vi "OE2012&OE2022_Ethernet_Query Data.vi"(0 "Connection ID in":refnum<k5>, 9 "Timeout":u32=40, 11 "Error in (no error)":errorcluster caption="error out（no error）") -> (1 "ChannelA_Configure":T1={"InputSource"=0, "InputCoupling"=0, "Input Range"=0, "Time Constant(s) "=0.0, "Low Pass Filter Slope "=1, "InputGround"=0, "Enable Sync Filter"=0, "Reference Source"=0, "External Ref Trigger"=0, "Phase0 (degree)"=0.0, "Phase1 (degree)"=0.0, "Phase2 (degree)"=0.0, "Phase3 (degree)"=0.0, "Phase4 (degree)"=0.0, "Phase5 (degree)"=0.0, "Phase6 (degree)"=0.0, "Phase7 (degree)"=0.0, "Osc1 Frequency(Hz)"=0.0, "Osc2 Frequency(Hz)"=0.0, "Demodulator type_1"=0, "Demodulator type_2"=0, "Demodulator type_3"=0, "Demodulator type_4"=0, "Demodulator type_5"=0, "Demodulator type_6"=0, "Demodulator type_7"=0, "Demodulator type_8"=0, "Demodulator harm_1"=0, "Demodulator harm_2"=0, "Demodulator harm_3"=0, "Demodulator harm_4"=0, "Demodulator harm_5"=0, "Demodulator harm_6"=0, "Demodulator harm_7"=0, "Demodulator harm_8"=0, "Demodulator freq_1"=0.0, "Demodulator freq_2"=0.0, "Demodulator freq_3"=0.0, "Demodulator freq_4"=0.0, "Demodulator freq_5"=0.0, "Demodulator freq_6"=0.0, "Demodulator freq_7"=0.0, "Demodulator freq_8"=0.0, "SineOut Mode"=0, "SineOut TTL Switch"=0, "Sine Output Amplitude(V)"=0.0, "Sine Output Offest (V)"=0.0, "CH1_Source"=3, "CH2_Source"=3, "CH3_Source"=3, "CH4_Source"=3, "CH1 AUX OUT"=0.0, "CH2 AUX OUT"=0.0, "CH3 AUX OUT"=0.0, "CH4 AUX OUT"=0.0, "CH1 Offset(%)"=0.0, "CH2 Offset(%)"=0.0, "CH3 Offset(%)"=0.0, "CH4 Offset(%)"=0.0, "CH1 Expand"=0.0, "CH2 Expand"=0.0, "CH3 Expand"=0.0, "CH4 Expand"=0.0, "CH1_Sensitivity "=24, "CH2_Sensitivity "=24, "CH3_Sensitivity"=24, "CH4_Sensitivity"=24, "Input ovld state"=FALSE, "Gain ovld state"=FALSE, "PLL state"=FALSE} {"CH4_Sensitivity" items=["1 nV/fA", "2 nV/fA", "5 nV/fA", "10 nV/fA", "20 nV/fA", "50 nV/fA", "100 nV/fA", "200 nV/fA", "500 nV/fA", "1 uV/pA", "2 uV/pA", "5 uV/pA", "10 uV/pA", "20 uV/pA", "50 uV/pA", "100 uV/pA", "200 uV/pA", "500 uV/pA", "1 mV/nA", "2 mV/nA", "5 mV/nA", "10 mV/nA", "20 mV/nA", "50 mV/nA", "100 mV/nA", "200 mV/nA", "500 mV/nA", "1 V/uA", "2 V/uA", "5 V/uA"]; "CH3_Sensitivity" items=["1 nV/fA", "2 nV/fA", "5 nV/fA", "10 nV/fA", "20 nV/fA", "50 nV/fA", "100 nV/fA", "200 nV/fA", "500 nV/fA", "1 uV/pA", "2 uV/pA", "5 uV/pA", "10 uV/pA", "20 uV/pA", "50 uV/pA", "100 uV/pA", "200 uV/pA", "500 uV/pA", "1 mV/nA", "2 mV/nA", "5 mV/nA", "10 mV/nA", "20 mV/nA", "50 mV/nA", "100 mV/nA", "200 mV/nA", "500 mV/nA", "1 V/uA", "2 V/uA", "5 V/uA"]; "CH2_Sensitivity" items=["1 nV/fA", "2 nV/fA", "5 nV/fA", "10 nV/fA", "20 nV/fA", "50 nV/fA", "100 nV/fA", "200 nV/fA", "500 nV/fA", "1 uV/pA", "2 uV/pA", "5 uV/pA", "10 uV/pA", "20 uV/pA", "50 uV/pA", "100 uV/pA", "200 uV/pA", "500 uV/pA", "1 mV/nA", "2 mV/nA", "5 mV/nA", "10 mV/nA", "20 mV/nA", "50 mV/nA", "100 mV/nA", "200 mV/nA", "500 mV/nA", "1 V/uA", "2 V/uA", "5 V/uA"]; "CH1_Sensitivity" items=["1 nV/fA", "2 nV/fA", "5 nV/fA", "10 nV/fA", "20 nV/fA", "50 nV/fA", "100 nV/fA", "200 nV/fA", "500 nV/fA", "1 uV/pA", "2 uV/pA", "5 uV/pA", "10 uV/pA", "20 uV/pA", "50 uV/pA", "100 uV/pA", "200 uV/pA", "500 uV/pA", "1 mV/nA", "2 mV/nA", "5 mV/nA", "10 mV/nA", "20 mV/nA", "50 mV/nA", "100 mV/nA", "200 mV/nA", "500 mV/nA", "1 V/uA", "2 V/uA", "5 V/uA"]; "CH4_Source" items=["DC OUT", "X-Demod1", "Y-Demod1", "R-Demod1", "Theta-Demod1", "X-Demod2", "Y-Demod2", "R-Demod2", "Theta-Demod2", "X-Demod3", "Y-Demod3", "R-Demod3", "Theta-Demod3", "X-Demod4", "Y-Demod4", "R-Demod4", "Theta-Demod4", "X-Demod5", "Y-Demod5", "R-Demod5", "Theta-Demod5", "X-Demod6", "Y-Demod6", "R-Demod6", "Theta-Demod6", "X-Demod7", "Y-Demod7", "R-Demod7", "Theta-Demod7", "X-Demod8", "Y-Demod8", "R-Demod8", "Theta-Demod8", "AUXIN1", "AUXIN2", "AUXIN3", "AUXIN4"]; "CH3_Source" items=["DC OUT", "X-Demod1", "Y-Demod1", "R-Demod1", "Theta-Demod1", "X-Demod2", "Y-Demod2", "R-Demod2", "Theta-Demod2", "X-Demod3", "Y-Demod3", "R-Demod3", "Theta-Demod3", "X-Demod4", "Y-Demod4", "R-Demod4", "Theta-Demod4", "X-Demod5", "Y-Demod5", "R-Demod5", "Theta-Demod5", "X-Demod6", "Y-Demod6", "R-Demod6", "Theta-Demod6", "X-Demod7", "Y-Demod7", "R-Demod7", "Theta-Demod7", "X-Demod8", "Y-Demod8", "R-Demod8", "Theta-Demod8", "AUXIN1", "AUXIN2", "AUXIN3", "AUXIN4"]; "CH2_Source" items=["DC OUT", "X-Demod1", "Y-Demod1", "R-Demod1", "Theta-Demod1", "X-Demod2", "Y-Demod2", "R-Demod2", "Theta-Demod2", "X-Demod3", "Y-Demod3", "R-Demod3", "Theta-Demod3", "X-Demod4", "Y-Demod4", "R-Demod4", "Theta-Demod4", "X-Demod5", "Y-Demod5", "R-Demod5", "Theta-Demod5", "X-Demod6", "Y-Demod6", "R-Demod6", "Theta-Demod6", "X-Demod7", "Y-Demod7", "R-Demod7", "Theta-Demod7", "X-Demod8", "Y-Demod8", "R-Demod8", "Theta-Demod8", "AUXIN1", "AUXIN2", "AUXIN3", "AUXIN4"]; "CH1_Source" items=["DC OUT", "X-Demod1", "Y-Demod1", "R-Demod1", "Theta-Demod1", "X-Demod2", "Y-Demod2", "R-Demod2", "Theta-Demod2", "X-Demod3", "Y-Demod3", "R-Demod3", "Theta-Demod3", "X-Demod4", "Y-Demod4", "R-Demod4", "Theta-Demod4", "X-Demod5", "Y-Demod5", "R-Demod5", "Theta-Demod5", "X-Demod6", "Y-Demod6", "R-Demod6", "Theta-Demod6", "X-Demod7", "Y-Demod7", "R-Demod7", "Theta-Demod7", "X-Demod8", "Y-Demod8", "R-Demod8", "Theta-Demod8", "AUXIN1", "AUXIN2", "AUXIN3", "AUXIN4"]; "SineOut TTL Switch" items=["OFF", "On"]; "SineOut Mode" items=["OFF", "On"]; "Demodulator type_8" items=["Osc1", "Osc2", "Harm", "Arb_Freq"]; "Demodulator type_7" items=["Osc1", "Osc2", "Harm", "Arb_Freq"]; "Demodulator type_6" items=["Osc1", "Osc2", "Harm", "Arb_Freq"]; "Demodulator type_5" items=["Osc1", "Osc2", "Harm", "Arb_Freq"]; "Demodulator type_4" items=["Osc1", "Osc2", "Harm", "Arb_Freq"]; "Demodulator type_3" items=["Osc1", "Osc2", "Harm", "Arb_Freq"]; "Demodulator type_2" items=["Osc1", "Osc2", "Harm", "Arb_Freq"]; "Demodulator type_1" items=["Osc1", "Osc2", "Harm", "Arb_Freq"]; "External Ref Trigger" items=["TTL Rising Edge", "TTL Fallling Edge", "Sine Zero Crossing"]; "Reference Source" items=["External", "Internal"]; "Enable Sync Filter" items=["OFF", "ON"]; "InputGround" items=["FLoat", "Ground"]; "Low Pass Filter Slope" items=["6 dB/oct", "12 dB/oct", "18 db/oct", "24 dB/oct", "30 dB/oct", "36 dB/oct", "42 dB/oct", "48 dB/oct"]; "Input Range" items=["2V", "500mV", "200mV", "50mV", "20mV", "5mV", "2mV"]; "InputCoupling" items=["AC", "DC"]; "InputSource" items=["A", "A-B", "Current"]}, 3 "Buffer Count":u8, 4 "Connection ID out":refnum<k5>, 6 "Parameter Values":T2, 8 "Total Date Array":dbl[][](array[numeric]), 10 "Output String":string, 12 "ChannelB_Configure":T1={"InputSource"=0, "InputCoupling"=0, "Input Range"=0, "Time Constant(s) "=0.0, "Low Pass Filter Slope "=1, "InputGround"=0, "Enable Sync Filter"=0, "Reference Source"=0, "External Ref Trigger"=0, "Phase0 (degree)"=0.0, "Phase1 (degree)"=0.0, "Phase2 (degree)"=0.0, "Phase3 (degree)"=0.0, "Phase4 (degree)"=0.0, "Phase5 (degree)"=0.0, "Phase6 (degree)"=0.0, "Phase7 (degree)"=0.0, "Osc1 Frequency(Hz)"=0.0, "Osc2 Frequency(Hz)"=0.0, "Demodulator type_1"=0, "Demodulator type_2"=0, "Demodulator type_3"=0, "Demodulator type_4"=0, "Demodulator type_5"=0, "Demodulator type_6"=0, "Demodulator type_7"=0, "Demodulator type_8"=0, "Demodulator harm_1"=0, "Demodulator harm_2"=0, "Demodulator harm_3"=0, "Demodulator harm_4"=0, "Demodulator harm_5"=0, "Demodulator harm_6"=0, "Demodulator harm_7"=0, "Demodulator harm_8"=0, "Demodulator freq_1"=0.0, "Demodulator freq_2"=0.0, "Demodulator freq_3"=0.0, "Demodulator freq_4"=0.0, "Demodulator freq_5"=0.0, "Demodulator freq_6"=0.0, "Demodulator freq_7"=0.0, "Demodulator freq_8"=0.0, "SineOut Mode"=0, "SineOut TTL Switch"=0, "Sine Output Amplitude(V)"=0.0, "Sine Output Offest (V)"=0.0, "CH1_Source"=3, "CH2_Source"=3, "CH3_Source"=3, "CH4_Source"=3, "CH1 AUX OUT"=0.0, "CH2 AUX OUT"=0.0, "CH3 AUX OUT"=0.0, "CH4 AUX OUT"=0.0, "CH1 Offset(%)"=0.0, "CH2 Offset(%)"=0.0, "CH3 Offset(%)"=0.0, "CH4 Offset(%)"=0.0, "CH1 Expand"=0.0, "CH2 Expand"=0.0, "CH3 Expand"=0.0, "CH4 Expand"=0.0, "CH1_Sensitivity "=24, "CH2_Sensitivity "=24, "CH3_Sensitivity"=24, "CH4_Sensitivity"=24, "Input ovld state"=FALSE, "Gain ovld state"=FALSE, "PLL state"=FALSE} {"CH4_Sensitivity" items=["1 nV/fA", "2 nV/fA", "5 nV/fA", "10 nV/fA", "20 nV/fA", "50 nV/fA", "100 nV/fA", "200 nV/fA", "500 nV/fA", "1 uV/pA", "2 uV/pA", "5 uV/pA", "10 uV/pA", "20 uV/pA", "50 uV/pA", "100 uV/pA", "200 uV/pA", "500 uV/pA", "1 mV/nA", "2 mV/nA", "5 mV/nA", "10 mV/nA", "20 mV/nA", "50 mV/nA", "100 mV/nA", "200 mV/nA", "500 mV/nA", "1 V/uA", "2 V/uA", "5 V/uA"]; "CH3_Sensitivity" items=["1 nV/fA", "2 nV/fA", "5 nV/fA", "10 nV/fA", "20 nV/fA", "50 nV/fA", "100 nV/fA", "200 nV/fA", "500 nV/fA", "1 uV/pA", "2 uV/pA", "5 uV/pA", "10 uV/pA", "20 uV/pA", "50 uV/pA", "100 uV/pA", "200 uV/pA", "500 uV/pA", "1 mV/nA", "2 mV/nA", "5 mV/nA", "10 mV/nA", "20 mV/nA", "50 mV/nA", "100 mV/nA", "200 mV/nA", "500 mV/nA", "1 V/uA", "2 V/uA", "5 V/uA"]; "CH2_Sensitivity" items=["1 nV/fA", "2 nV/fA", "5 nV/fA", "10 nV/fA", "20 nV/fA", "50 nV/fA", "100 nV/fA", "200 nV/fA", "500 nV/fA", "1 uV/pA", "2 uV/pA", "5 uV/pA", "10 uV/pA", "20 uV/pA", "50 uV/pA", "100 uV/pA", "200 uV/pA", "500 uV/pA", "1 mV/nA", "2 mV/nA", "5 mV/nA", "10 mV/nA", "20 mV/nA", "50 mV/nA", "100 mV/nA", "200 mV/nA", "500 mV/nA", "1 V/uA", "2 V/uA", "5 V/uA"]; "CH1_Sensitivity" items=["1 nV/fA", "2 nV/fA", "5 nV/fA", "10 nV/fA", "20 nV/fA", "50 nV/fA", "100 nV/fA", "200 nV/fA", "500 nV/fA", "1 uV/pA", "2 uV/pA", "5 uV/pA", "10 uV/pA", "20 uV/pA", "50 uV/pA", "100 uV/pA", "200 uV/pA", "500 uV/pA", "1 mV/nA", "2 mV/nA", "5 mV/nA", "10 mV/nA", "20 mV/nA", "50 mV/nA", "100 mV/nA", "200 mV/nA", "500 mV/nA", "1 V/uA", "2 V/uA", "5 V/uA"]; "CH4_Source" items=["DC OUT", "X-Demod1", "Y-Demod1", "R-Demod1", "Theta-Demod1", "X-Demod2", "Y-Demod2", "R-Demod2", "Theta-Demod2", "X-Demod3", "Y-Demod3", "R-Demod3", "Theta-Demod3", "X-Demod4", "Y-Demod4", "R-Demod4", "Theta-Demod4", "X-Demod5", "Y-Demod5", "R-Demod5", "Theta-Demod5", "X-Demod6", "Y-Demod6", "R-Demod6", "Theta-Demod6", "X-Demod7", "Y-Demod7", "R-Demod7", "Theta-Demod7", "X-Demod8", "Y-Demod8", "R-Demod8", "Theta-Demod8", "AUXIN1", "AUXIN2", "AUXIN3", "AUXIN4"]; "CH3_Source" items=["DC OUT", "X-Demod1", "Y-Demod1", "R-Demod1", "Theta-Demod1", "X-Demod2", "Y-Demod2", "R-Demod2", "Theta-Demod2", "X-Demod3", "Y-Demod3", "R-Demod3", "Theta-Demod3", "X-Demod4", "Y-Demod4", "R-Demod4", "Theta-Demod4", "X-Demod5", "Y-Demod5", "R-Demod5", "Theta-Demod5", "X-Demod6", "Y-Demod6", "R-Demod6", "Theta-Demod6", "X-Demod7", "Y-Demod7", "R-Demod7", "Theta-Demod7", "X-Demod8", "Y-Demod8", "R-Demod8", "Theta-Demod8", "AUXIN1", "AUXIN2", "AUXIN3", "AUXIN4"]; "CH2_Source" items=["DC OUT", "X-Demod1", "Y-Demod1", "R-Demod1", "Theta-Demod1", "X-Demod2", "Y-Demod2", "R-Demod2", "Theta-Demod2", "X-Demod3", "Y-Demod3", "R-Demod3", "Theta-Demod3", "X-Demod4", "Y-Demod4", "R-Demod4", "Theta-Demod4", "X-Demod5", "Y-Demod5", "R-Demod5", "Theta-Demod5", "X-Demod6", "Y-Demod6", "R-Demod6", "Theta-Demod6", "X-Demod7", "Y-Demod7", "R-Demod7", "Theta-Demod7", "X-Demod8", "Y-Demod8", "R-Demod8", "Theta-Demod8", "AUXIN1", "AUXIN2", "AUXIN3", "AUXIN4"]; "CH1_Source" items=["DC OUT", "X-Demod1", "Y-Demod1", "R-Demod1", "Theta-Demod1", "X-Demod2", "Y-Demod2", "R-Demod2", "Theta-Demod2", "X-Demod3", "Y-Demod3", "R-Demod3", "Theta-Demod3", "X-Demod4", "Y-Demod4", "R-Demod4", "Theta-Demod4", "X-Demod5", "Y-Demod5", "R-Demod5", "Theta-Demod5", "X-Demod6", "Y-Demod6", "R-Demod6", "Theta-Demod6", "X-Demod7", "Y-Demod7", "R-Demod7", "Theta-Demod7", "X-Demod8", "Y-Demod8", "R-Demod8", "Theta-Demod8", "AUXIN1", "AUXIN2", "AUXIN3", "AUXIN4"]; "SineOut TTL Switch" items=["OFF", "On"]; "SineOut Mode" items=["OFF", "On"]; "Demodulator type_8" items=["Osc1", "Osc2", "Harm", "Arb_Freq"]; "Demodulator type_7" items=["Osc1", "Osc2", "Harm", "Arb_Freq"]; "Demodulator type_6" items=["Osc1", "Osc2", "Harm", "Arb_Freq"]; "Demodulator type_5" items=["Osc1", "Osc2", "Harm", "Arb_Freq"]; "Demodulator type_4" items=["Osc1", "Osc2", "Harm", "Arb_Freq"]; "Demodulator type_3" items=["Osc1", "Osc2", "Harm", "Arb_Freq"]; "Demodulator type_2" items=["Osc1", "Osc2", "Harm", "Arb_Freq"]; "Demodulator type_1" items=["Osc1", "Osc2", "Harm", "Arb_Freq"]; "External Ref Trigger" items=["TTL Rising Edge", "TTL Fallling Edge", "Sine Zero Crossing"]; "Reference Source" items=["External", "Internal"]; "Enable Sync Filter" items=["OFF", "ON"]; "InputGround" items=["FLoat", "Ground"]; "Low Pass Filter Slope" items=["6 dB/oct", "12 dB/oct", "18 db/oct", "24 dB/oct", "30 dB/oct", "36 dB/oct", "42 dB/oct", "48 dB/oct"]; "Input Range" items=["2V", "500mV", "200mV", "50mV", "20mV", "5mV", "2mV"]; "InputCoupling" items=["AC", "DC"]; "InputSource" items=["A", "A-B", "Current"]}, 13 "Trig_Count":u8[](array[numeric]), 14 "PLL&Overload":T3, 15 "Error out":errorcluster caption="error out")   [LabVIEW 2011]
panel:
  out "Read Buffer":string
  in  "buffer":string
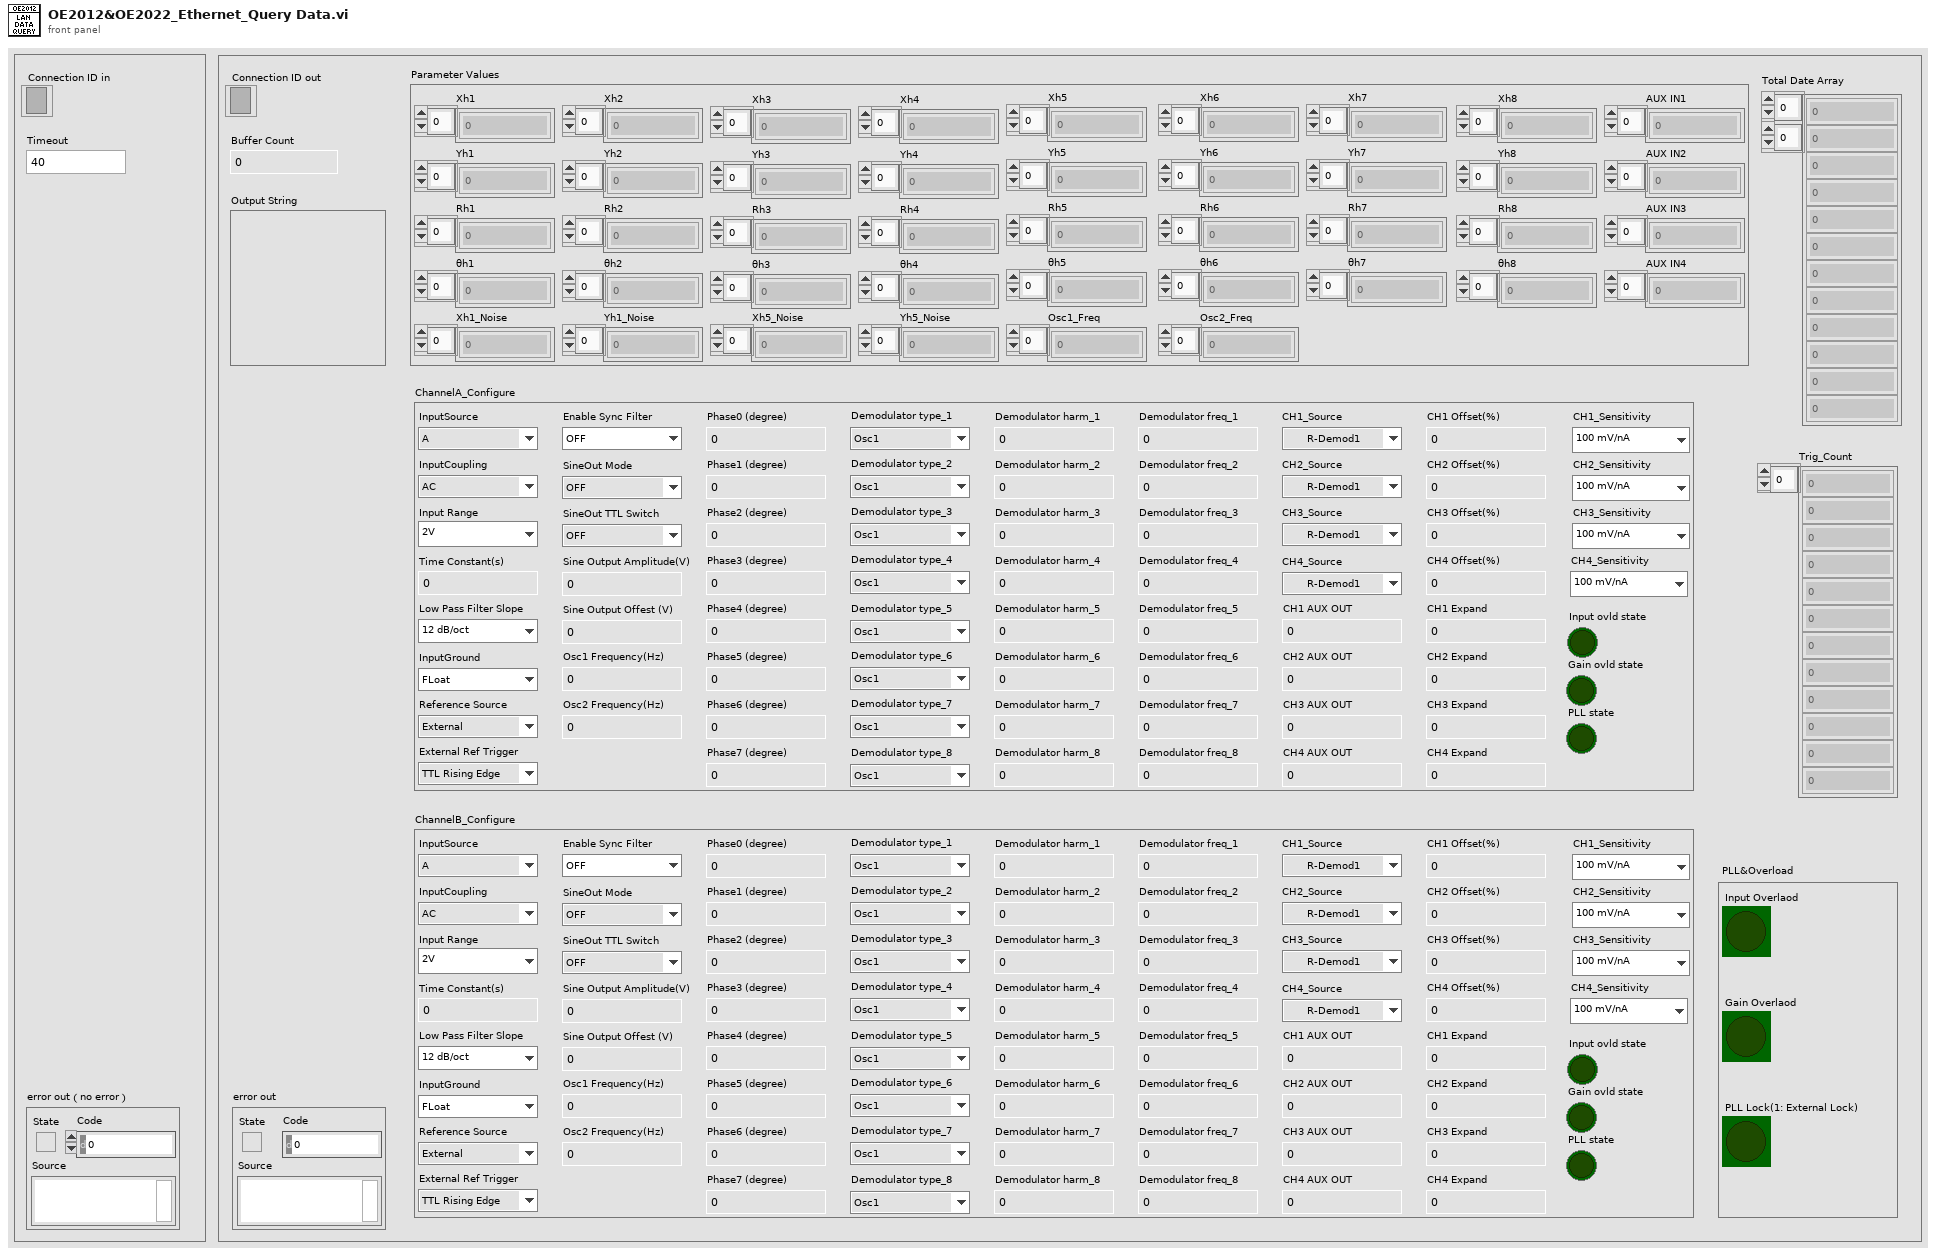
[diagram p1: front panel]
types:
  T1 = cluster{"InputSource":u8, "InputCoupling":u8, "Input Range":u8, "Time Constant(s) ":dbl, "Low Pass Filter Slope ":u8, "InputGround":u8, "Enable Sync Filter":u8, "Reference Source":u8, "External Ref Trigger":u8, "Phase0 (degree)":sgl, "Phase1 (degree)":sgl, "Phase2 (degree)":sgl, "Phase3 (degree)":sgl, "Phase4 (degree)":sgl, "Phase5 (degree)":sgl, "Phase6 (degree)":sgl, "Phase7 (degree)":sgl, "Osc1 Frequency(Hz)":dbl, "Osc2 Frequency(Hz)":dbl, "Demodulator type_1":u8, "Demodulator type_2":u8, "Demodulator type_3":u8, "Demodulator type_4":u8, "Demodulator type_5":u8, "Demodulator type_6":u8, "Demodulator type_7":u8, "Demodulator type_8":u8, "Demodulator harm_1":u16, "Demodulator harm_2":u16, "Demodulator harm_3":u16, "Demodulator harm_4":u16, "Demodulator harm_5":u16, "Demodulator harm_6":u16, "Demodulator harm_7":u16, "Demodulator harm_8":u16, "Demodulator freq_1":dbl, "Demodulator freq_2":dbl, "Demodulator freq_3":dbl, "Demodulator freq_4":dbl, "Demodulator freq_5":dbl, "Demodulator freq_6":dbl, "Demodulator freq_7":dbl, "Demodulator freq_8":dbl, "SineOut Mode":u8, "SineOut TTL Switch":u8, "Sine Output Amplitude(V)":dbl, "Sine Output Offest (V)":dbl, "CH1_Source":u8, "CH2_Source":u8, "CH3_Source":u8, "CH4_Source":u8, "CH1 AUX OUT":dbl, "CH2 AUX OUT":dbl, "CH3 AUX OUT":dbl, "CH4 AUX OUT":dbl, "CH1 Offset(%)":dbl, "CH2 Offset(%)":dbl, "CH3 Offset(%)":dbl, "CH4 Offset(%)":dbl, "CH1 Expand":dbl, "CH2 Expand":dbl, "CH3 Expand":dbl, "CH4 Expand":dbl, "CH1_Sensitivity ":u8, "CH2_Sensitivity ":u8, "CH3_Sensitivity":u8, "CH4_Sensitivity":u8, "Input ovld state":bool, "Gain ovld state":bool, "PLL state":bool}
  T2 = cluster{"Xh1":dbl[], "Yh1":dbl[], "Rh1":dbl[], "θh1":dbl[], "Xh1_Noise":dbl[], "Yh1_Noise":dbl[], "Xh2":dbl[], "Yh2":dbl[], "Rh2":dbl[], "θh2":dbl[], "Xh3":dbl[], "Yh3":dbl[], "Rh3":dbl[], "θh3":dbl[], "Xh4":dbl[], "Yh4":dbl[], "Rh4":dbl[], "θh4":dbl[], "Xh5":dbl[], "Yh5":dbl[], "Rh5":dbl[], "θh5":dbl[], "Xh5_Noise":dbl[], "Yh5_Noise":dbl[], "Xh6":dbl[], "Yh6":dbl[], "Rh6":dbl[], "θh6":dbl[], "Xh7":dbl[], "Yh7":dbl[], "Rh7":dbl[], "θh7":dbl[], "Xh8":dbl[], "Yh8":dbl[], "Rh8":dbl[], "θh8":dbl[], "Osc1_Freq":dbl[], "Osc2_Freq":dbl[], "AUX IN1":dbl[], "AUX IN2":dbl[], "AUX IN3":dbl[], "AUX IN4":dbl[]}
  T3 = cluster{"Input Overlaod":bool, "Gain Overlaod":bool, "PLL Lock(1: External Lock)":bool}
  T4 = cluster{"Xh1":dbl[], "Yh1":dbl[], "Rh1":dbl[], "θh1":dbl[], "Xh1_Noise":dbl[], "Yh1_Noise":dbl[], "Xh2":dbl[], "Yh2":dbl[], "Rh2":dbl[], "θh2":dbl[], "Xh3":dbl[], "Yh3":dbl[], "Rh3":dbl[], "θh3":dbl[], "Xh4":dbl[], "Yh4":dbl[], "Rh4":dbl[], "θh4":dbl[], "Xh5":dbl[], "Yh5":dbl[], "Rh5":dbl[], "θh5":dbl[], "Xh5_Noise":dbl[], "Yh5_Noise":dbl[], "Xh6":dbl[], "Yh6":dbl[], "Rh6":dbl[], "θh6":dbl[], "Xh7":dbl[], "Yh7":dbl[], "Rh7":dbl[], "θh7":dbl[], "Xh8":dbl[], "Yh8":dbl[], "Rh8":dbl[], "θh8":dbl[], "Osc1_Freq":dbl[], "Osc2_Freq":dbl[], "AUXOUT1":dbl[], "AUXOUT2":dbl[], "AUXOUT3":dbl[], "AUXOUT4":dbl[]}
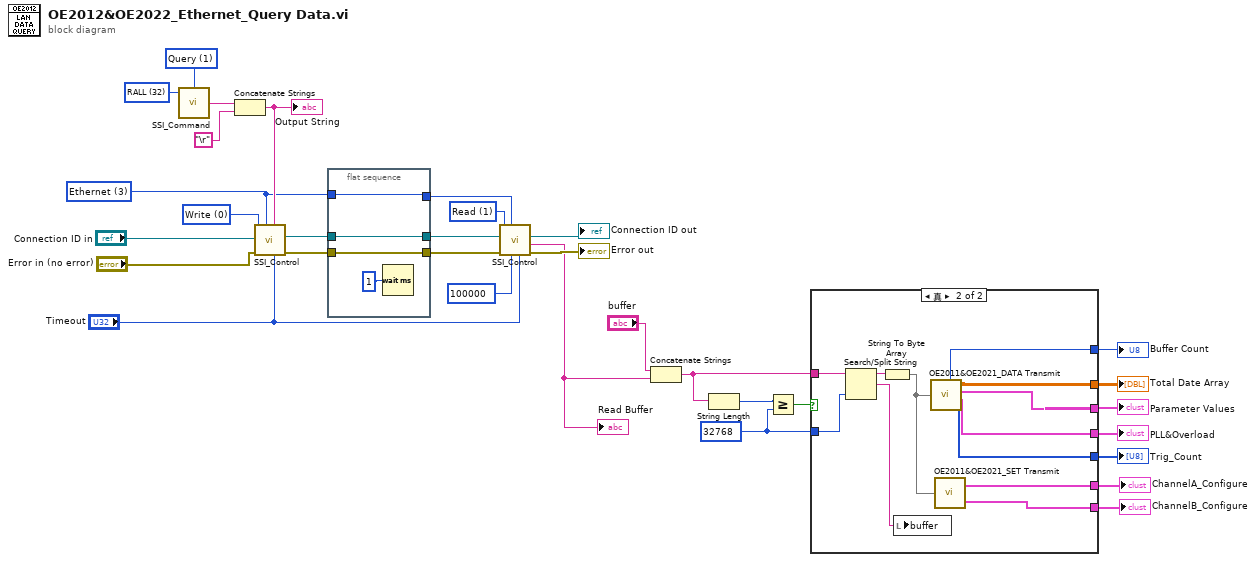
[diagram p0: block diagram]
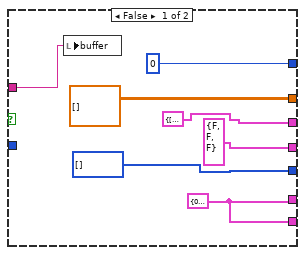
[diagram p2: hidden frame]
diagram:
  w9 = 32768 ("y")
  w26 = u16 3 items=["USB", "RS232", "GPIB", "Ethernet"] ("Remote Mode")
  w22 = u16 32 items=["ISRC", "IGND", "ICPL", "ILIN", "PHAS", "FMOD", "RSLP", "FREQ", "SWPT", "SLLM", "SULM", "SSLL", "SSLG", "STLM", "SWRM", "IRNG", "SENS", "RMOD", "OFLT", "OFSL", "SYNC", "DMOD", "HARM", "DARB", "SWVT", "SLVL", "SVLL", "SVUL", "SVSL", "SVSG", "SVTM", "SVRM", "RALL", "SNAP", "OUTP", "OAUX", "COUT", "CAUX", "COFP", "CEXP", "FPOP", "OEXP", "*IDN", "*RST", "OVLD", "INOV", "GNOV", "*PLL", "SSET", "RSET", "AGAN", "APHS", "ARSV", "ASCL", "EQCD", "EQCS", "SPED", "SRAT", "SLEN", "SSLE", "STRG", "SPRM", "STRD", "PAUS", "RSET", "SPTS", "TRCA", "TEMP", "RSTU", "INHZ", "DEQU", "SADD", "ARNG", "CSPE", "ISRCD", "IGNDD", "ICPLD", "ILIND", "PHASD", "FMODD", "RSLPD", "FREQD", "SWPTD", "SLLMD", "SULMD", "SSLLD", "SSLGD", "STLMD", "SWRMD", "SENSD", "RMODD", "OFLTD", "OFSLD", "SYNCD", "HARMD", "EQCDD", "EQCSD", "SNAPD", "OUTPD", "SWVTD", "SLVLD", "SVLLD", "SVULD", "SVSLD", "SVSGD", "SVTMD", "SVRMD", "SVDCD", "ARSVD", "AGAND", "APHSD", "ASCLD", "FPOPD", "CAUXD", "OEXPD", "SPEDD", "SRATD", "SLEND", "SSLED", "STRGD", "SPRMD", "STRDD", "PAUSD", "RESTD", "SPTSD", "TRCAD", "*IDND", "*RSTD", "INOVD", "GNOVD", "*PLLD", "SSETD", "RSETD", "RALLD"] ("Command Type")
  w20 = u16 1 items=["Set", "Query"] ("Opera")
  w29 = u16 1 items=["Write", "Read"] ("Control")
  w32 = u16 0 items=["Write", "Read"] ("Control")
  n1 = call "SSI_Command.vi"("Opera"=w20, "Command Type"=w22) -> ("Output string"=w21:string)  [unwired: 2 in]
  n2 = Concatenate Strings(w21, "\r") -> (w27:string)
  "Output String" <- w27
  n3 = call "SSI_Control.vi"("Tineout"="Timeout", "Write Buffer"=w27, "Remote Mode"=w26, "Error in (no error)"="Error in (no error)", "Control"=w32, "Connection ID in"="Connection ID in") -> ("Error out"=w31:errorcluster, "Connection ID out"=w6:refnum<k5>)  [unwired: 2 in, 2 out]
  n4 = flat-sequence {
    tunnel: w31 -> [w36]
    tunnel: [w36] -> w30
    tunnel: [w34] -> w28
    tunnel: w26 -> [w34]
    tunnel: w6 -> [w33]
    tunnel: [w33] -> w5
    frame #0 {
      n5 = Wait (ms)(milliseconds to wait=u32 1 ("等待时间（毫秒）")) -> ()  [unwired: 1 out]
    }
  }
  n6 = call "SSI_Control.vi"("Tineout"="Timeout", "Number of bytes"=u32 100000, "Remote Mode"=w28, "Error in (no error)"=w30, "Control"=w29, "Connection ID in"=w5) -> ("Error out"=→"Error out":errorcluster, "Read Buffer"=w4:string, "Connection ID out"=→"Connection ID out":refnum<k5>)  [unwired: 2 in, 1 out]
  "Read Buffer" <- w4
  n7 = Concatenate Strings("buffer", w4) -> (w12:string)
  n8 = String Length(string=w12) -> (length=w11:i32)
  n9 = Greater Or Equal?(x=w11, y=w9) -> (x >= y?=w19:bool)
  n10 = case shown="真" w19 {
    tunnel: [u8 0 w44] -> w17
    tunnel: [dbl[][] [] ("Total Data Array") w55] -> w16
    tunnel: [T3 {"Input Overlaod"=FALSE, "Gain Overlaod"=FALSE, "PLL Lock(1: External Lock)"=FALSE} ("PLL&Overload") w54] -> w15
    tunnel: [u8[] [] w53] -> w14
    tunnel: [T4 {"Xh1"=[], "Yh1"=[], "Rh1"=[], "θh1"=[], "Xh1_Noise"=[], "Yh1_Noise"=[], "Xh2"=[], "Yh2"=[], "Rh2"=[], "θh2"=[], "Xh3"=[], "Yh3"=[], "Rh3"=[], "θh3"=[], "Xh4"=[], "Yh4"=[], "Rh4"=[], "θh4"=[], "Xh5"=[], "Yh5"=[], "Rh5"=[], "θh5"=[], "Xh5_Noise"=[], "Yh5_Noise"=[], "Xh6"=[], "Yh6"=[], "Rh6"=[], "θh6"=[], "Xh7"=[], "Yh7"=[], "Rh7"=[], "θh7"=[], "Xh8"=[], "Yh8"=[], "Rh8"=[], "θh8"=[], "Osc1_Freq"=[], "Osc2_Freq"=[], "AUXOUT1"=[], "AUXOUT2"=[], "AUXOUT3"=[], "AUXOUT4"=[]} ("Parameter Values") w52] -> w13
    tunnel: w12 -> [w38 w50]
    tunnel: w9 -> [_ w48]
    tunnel: [w37 w46] -> w2
    tunnel: [w37 w45] -> w1
    frame False {
      w37 = T1 {"InputSource"=0, "InputCoupling"=0, "Input Range"=0, "Time Constant(s) "=0.0, "Low Pass Filter Slope "=0, "InputGround"=0, "Enable Sync Filter"=0, "Reference Source"=0, "External Ref Trigger"=0, "Phase0 (degree)"=0.0, "Phase1 (degree)"=0.0, "Phase2 (degree)"=0.0, "Phase3 (degree)"=0.0, "Phase4 (degree)"=0.0, "Phase5 (degree)"=0.0, "Phase6 (degree)"=0.0, "Phase7 (degree)"=0.0, "Osc1 Frequency(Hz)"=0.0, "Osc2 Frequency(Hz)"=0.0, "Demodulator type_1"=0, "Demodulator type_2"=0, "Demodulator type_3"=0, "Demodulator type_4"=0, "Demodulator type_5"=0, "Demodulator type_6"=0, "Demodulator type_7"=0, "Demodulator type_8"=0, "Demodulator harm_1"=0, "Demodulator harm_2"=0, "Demodulator harm_3"=0, "Demodulator harm_4"=0, "Demodulator harm_5"=0, "Demodulator harm_6"=0, "Demodulator harm_7"=0, "Demodulator harm_8"=0, "Demodulator freq_1"=0.0, "Demodulator freq_2"=0.0, "Demodulator freq_3"=0.0, "Demodulator freq_4"=0.0, "Demodulator freq_5"=0.0, "Demodulator freq_6"=0.0, "Demodulator freq_7"=0.0, "Demodulator freq_8"=0.0, "SineOut Mode"=0, "SineOut TTL Switch"=0, "Sine Output Amplitude(V)"=0.0, "Sine Output Offest (V)"=0.0, "CH1_Source"=0, "CH2_Source"=0, "CH3_Source"=0, "CH4_Source"=0, "CH1 AUX OUT"=0.0, "CH2 AUX OUT"=0.0, "CH3 AUX OUT"=0.0, "CH4 AUX OUT"=0.0, "CH1 Offset(%)"=0.0, "CH2 Offset(%)"=0.0, "CH3 Offset(%)"=0.0, "CH4 Offset(%)"=0.0, "CH1 Expand"=0.0, "CH2 Expand"=0.0, "CH3 Expand"=0.0, "CH4 Expand"=0.0, "CH1_Sensitivity "=0, "CH2_Sensitivity "=0, "CH3_Sensitivity"=0, "CH4_Sensitivity"=0, "Input ovld state"=FALSE, "Gain ovld state"=FALSE, "PLL state"=FALSE} ("ChannelA_Configure")
      n11 = local write "buffer"(w38) -> ()
    }
    frame True {
      n12 = Search/Split String(string=w50, offset (0)=w48) -> (substring before match=w51:string, match + rest of string=w49:string)  [unwired: 1 in, 1 out]
      n13 = String To Byte Array(string=w51) -> (unsigned byte array=w47:u8[])
      n14 = local write "buffer"(w49) -> ()
      n15 = call "OE2011&OE2021_DATA Transmit.vi"("Input Data"=w47) -> ("Trig_Count"=w53:u8[], "PLL&Overload"=w54:T3, "Parameter Values"=w52:T2, "Total Date Array"=w55:dbl[][], "Buffer Count"=w44:u8)
      n16 = call "OE2011&OE2021_SET Transmit.vi"("Input Data"=w47) -> ("ChannelA_Configure"=w46:T1, "ChannelB_Configure"=w45:T1)
    }
  }
  "Buffer Count" <- w17
  "Trig_Count" <- w14
  "PLL&Overload" <- w15
  "Total Date Array" <- w16
  "Parameter Values" <- w13
  "ChannelB_Configure" <- w1
  "ChannelA_Configure" <- w2
